vi "1C.1 Camera - find boat given marker locations.vi"(6 "Stern Marker Found":T1, 7 "Bow Marker Found":T1, 8 "Stern Marker Location":T3, 9 "Stern Marker Heading":T2 format="%05.1f", 10 "Bow Marker Location":T3, 11 "Bow Marker Heading":T2 format="%05.1f") -> (1 "Boat Found":T1, 2 "Heading":T2 format="%05.1f", 3 "Boat Location":T3)   [LabVIEW 2011]
doc: "Takes the information from two marker-finders, one for the bow and one for stern of the boat, and uses them to estimate the position of the center of the boat. \nAssumes that the center of the boat is either:\na. halfway in between the markers if both are found\nb. half of a boat length extrapolated in the appropriate direction from the marker that was found, if only one marker was found.\nIf neither marker was found, the Boat Found output will be False and you'll have to look elsewhere for your boat location information, sorry."
uses:
  2-RIO/2 Typedefs/UTM Location.ctl
  2-RIO/2 Typedefs/heading.ctl
  2-RIO/2 Typedefs/indicator LED.ctl
  2-RIO/2 Typedefs/Velocity.ctl
panel:
  in  "Distance Bow to Stern (m)":dbl=1.0
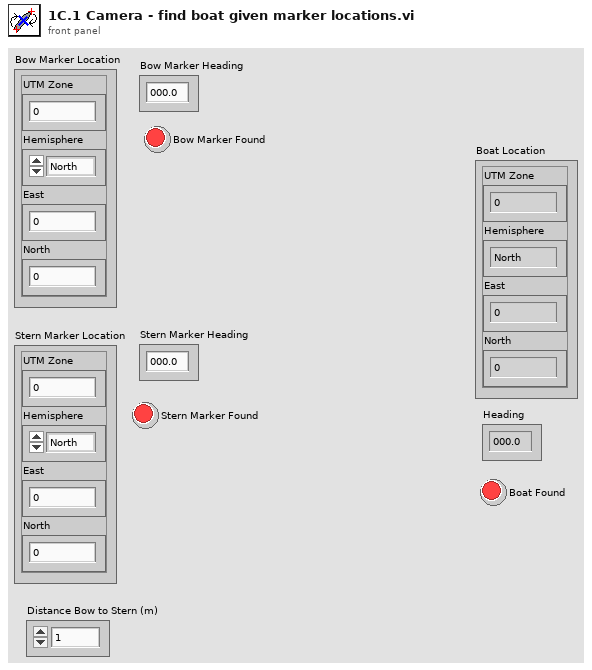
[diagram p1: front panel]
types:
  T1 = typedef "indicator LED.ctl" = bool
  T2 = typedef "heading.ctl" = dbl
  T3 = typedef "UTM Location.ctl" = cluster{"UTM Zone":dbl, "Hemisphere":enum16{"North", "South"}, "East":dbl, "North":dbl}
  T4 = typedef "Velocity.ctl" = cluster{"East":dbl, "North":dbl}
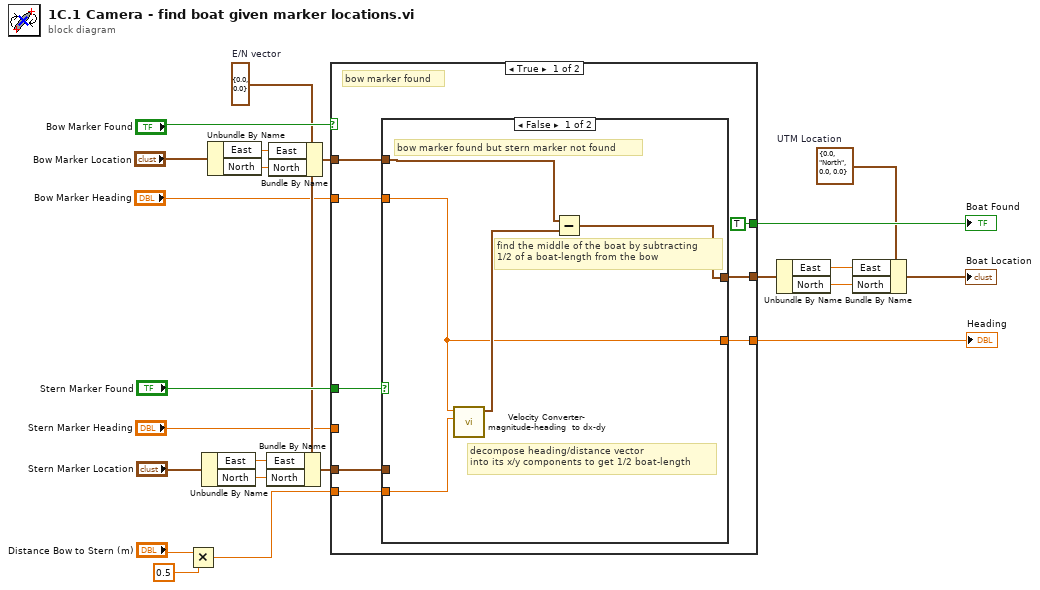
[diagram p0: block diagram]
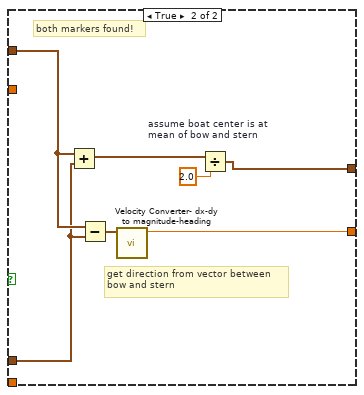
[diagram p2: hidden frame]
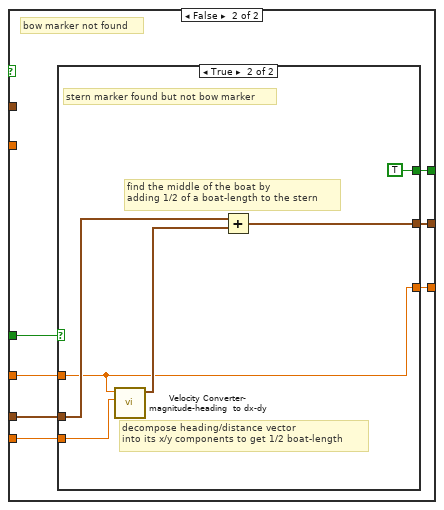
[diagram p3: hidden frame]
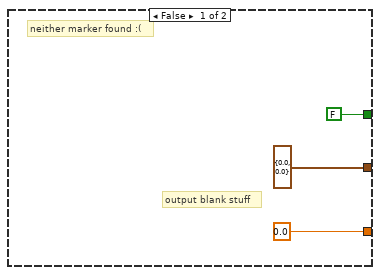
[diagram p4: hidden frame]
diagram:
  w7 = T3 {"UTM Zone"=0.0, "Hemisphere"=enum."North", "East"=0.0, "North"=0.0}  # UTM Location
  w11 = T4 {"East"=0.0, "North"=0.0}  # E/N vector
  n1 = Multiply(x="Distance Bow to Stern (m)", y=0.5) -> (x*y=w3:dbl)
  n2 = Unbundle By Name("Stern Marker Location") -> ("East"=w14:dbl, "North"=w13:dbl)
  n3 = Unbundle By Name("Bow Marker Location") -> ("East"=w16:dbl, "North"=w15:dbl)
  n4 = Bundle By Name(cluster=w11, "East"=w14, "North"=w13) -> (w12:T4)
  n5 = Bundle By Name(cluster=w11, "East"=w16, "North"=w15) -> (w17:T4)
  n6 = case shown="True" "Bow Marker Found" {
    tunnel: "Stern Marker Found" -> [w31 w50]
    tunnel: [TRUE w49] -> w21
    tunnel: [w27 w48] -> w20
    tunnel: w17 -> [w30 _]
    tunnel: w12 -> [w29 w44]
    tunnel: [w26 w47] -> w9
    tunnel: w3 -> [w25 w45]
    tunnel: "Bow Marker Heading" -> [w24 _]
    tunnel: "Stern Marker Heading" -> [_ w46]
    frame True {
      # "bow marker found"
      n7 = case shown="False" w31 {
        tunnel: w30 -> [w35 w41]
        tunnel: w29 -> [_ w40]
        tunnel: [w32 w42] -> w27
        tunnel: [w33 w37] -> w26
        tunnel: w25 -> [w36 _]
        tunnel: w24 -> [w32 _]
        frame False {
          # "decompose heading/distance vector \ninto its x/y components to get 1/2 boat-length"
          # "find the middle of the boat by subtracting \n1/2 of a boat-length from the bow"
          # "bow marker found but stern marker not found"
          n8 = call "Velocity Converter- magnitude-heading  to dx-dy.vi"("Magnitude"=w36, "Heading"=w32) -> ("Vector Out"=w34:T4)  [unwired: 9 in]
          n9 = Subtract(x=w35, y=w34) -> (x-y=w33:T4)
        }
        frame True {
          # "get direction from vector between\nbow and stern"
          # "both markers found!"
          n10 = Add(x=w41, y=w40) -> (x+y=w39:T4)
          n11 = Subtract(x=w41, y=w40) -> (x-y=w43:T4)
          n12 = call "Velocity Converter- dx-dy to magnitude-heading.vi"("Vector In"=w43) -> ("Heading Out"=w42:T2)  [unwired: 9 in, 1 out]
          n13 = Divide "assume boat center is at\nmean of bow and stern"(x=w39, y=2.0) -> (x/y=w37:T4)
        }
      }
    }
    frame False {
      # "bow marker not found"
      n14 = case shown="True" w50 {
        tunnel: [FALSE TRUE] -> w49
        tunnel: [T2 0.0 ("Heading") w54] -> w48
        tunnel: [T4 {"East"=0.0, "North"=0.0} ("E/N vector") w55] -> w47
        tunnel: w46 -> [_ w54]
        tunnel: w45 -> [_ w58]
        tunnel: w44 -> [_ w56]
        frame False {
          # "output blank stuff"
          # "neither marker found :("
        }
        frame True {
          # "find the middle of the boat by\nadding 1/2 of a boat-length to the stern"
          # "decompose heading/distance vector \ninto its x/y components to get 1/2 boat-length"
          # "stern marker found but not bow marker"
          n15 = call "Velocity Converter- magnitude-heading  to dx-dy.vi"("Magnitude"=w58, "Heading"=w54) -> ("Vector Out"=w57:T4)  [unwired: 9 in]
          n16 = Add(x=w56, y=w57) -> (x+y=w55:T4)
        }
      }
    }
  }
  "Heading" <- w20
  "Boat Found" <- w21
  n17 = Unbundle By Name(w9) -> ("East"=w10:dbl, "North"=w8:dbl)
  n18 = Bundle By Name(cluster=w7, "East"=w10, "North"=w8) -> (→"Boat Location":T3)
